vi "MFC-RT.vi"(0 "MFC":string(combo)="27", 5 "Set Point\n(SCCM)":dbl(knob) min=0.0 max=5000.0 step=1.0 scale=0.0..5000.0) -> ()   [LabVIEW 2011]
panel:
  out "SCCM":dbl=500.0
  in  "stop":bool
  in  "Full Scale":dbl=24576.0
  out "Pressure\n(%)":dbl(slide) scale=0.0..133.0
  out "Flow\n(SCCM)":dbl(slide) scale=0.0..6650.0
  out "Valve":i16
  out "Active Instance":i8
  out "Manufacturer Specific Warnings":bool caption="Boolean"
  out "Device Profice Specific Warnings":bool caption="Boolean"
  out "Common Warnings":bool caption="Boolean"
  out "0":bool caption="Boolean"
  out "Manufactuer Specific Alarms":bool caption="Boolean"
  out "1 (Extended Reporting Enabled)":bool caption="Boolean"
  out "Device Profile Specific Alarms":bool caption="Boolean"
  out "Common Alarms":bool caption="Boolean"
  # "0    -  24576\n   0% to  100%\n\n\n 24577  - 27033\n100+% to 110%\n\n\n 27034  -  32767\n110+% to 133%"
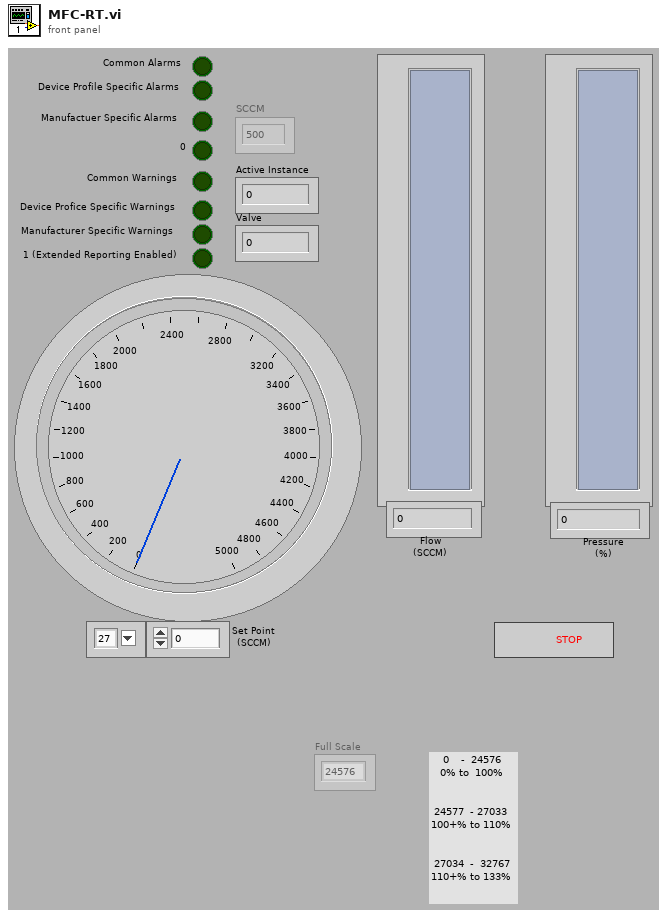
[diagram p1: front panel]
types:
  T1 = enum16{"No dialog", "OK message", "Continue or stop message", "OK message with warnings", "Continue or stop message with warnings"}
  T2 = enum16{"Read", "Write", "ReadWrite", "BufferedRead", "BufferedReadWrite"}
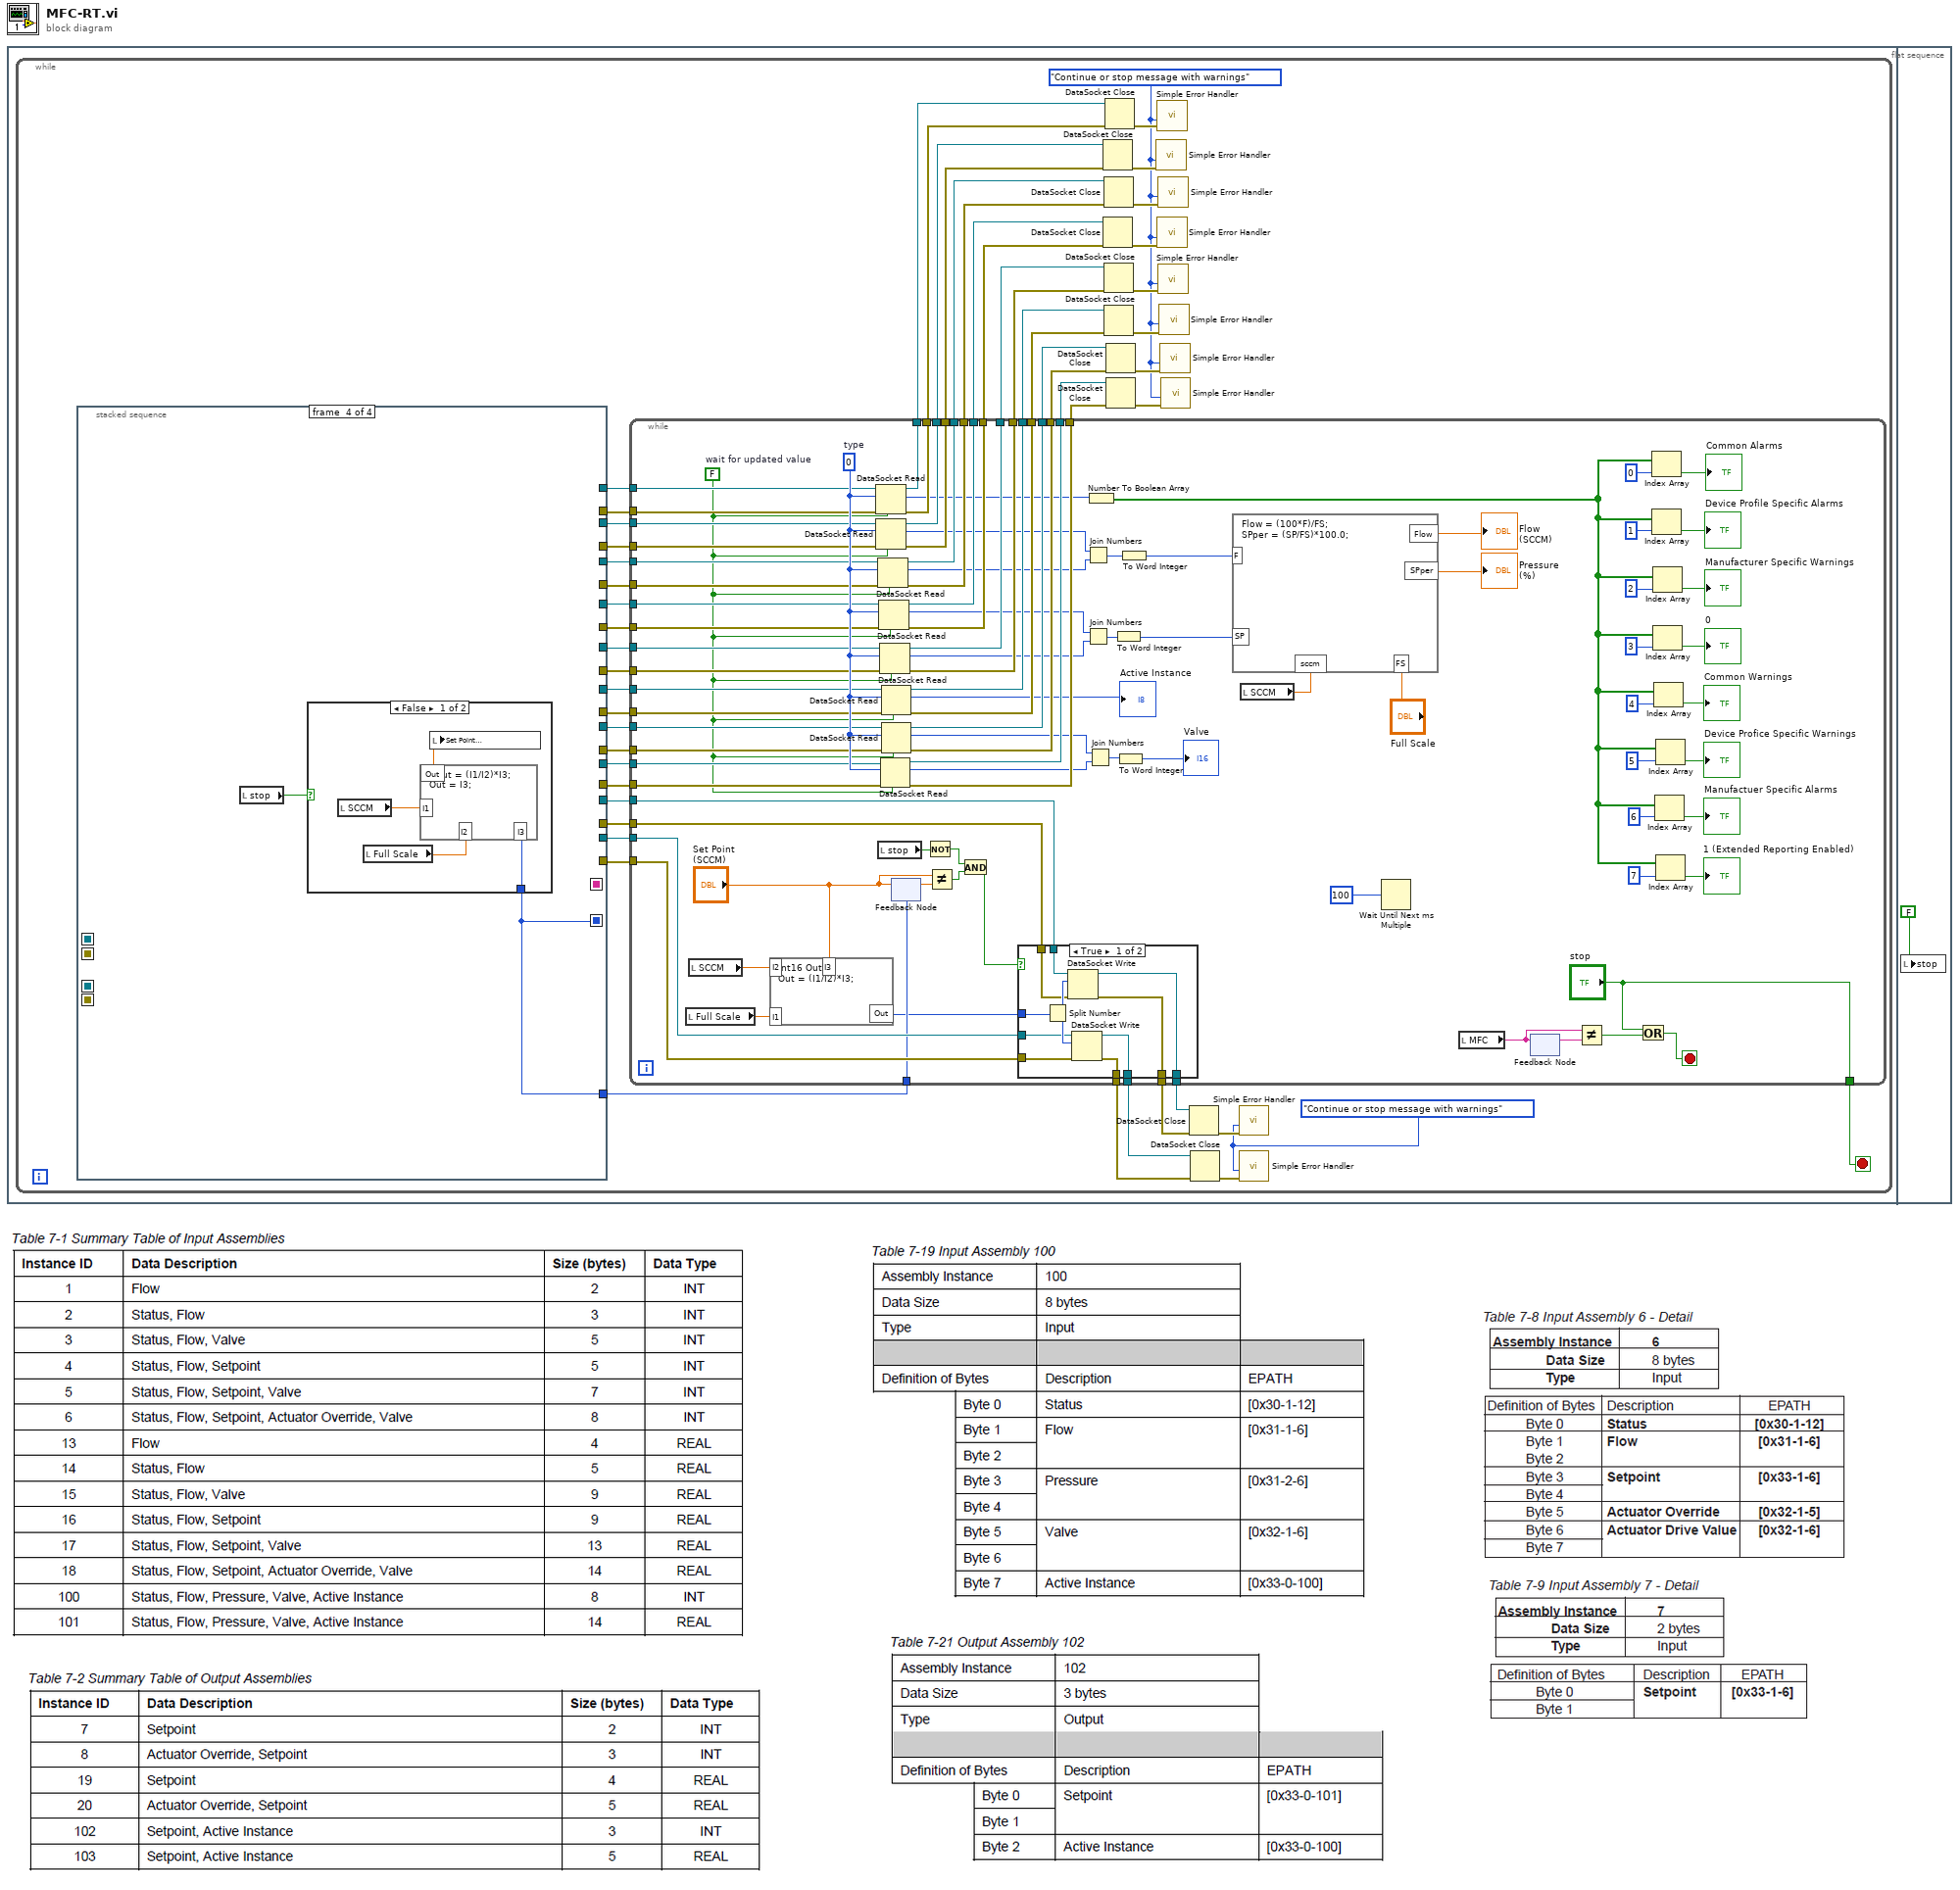
[diagram p0: block diagram]
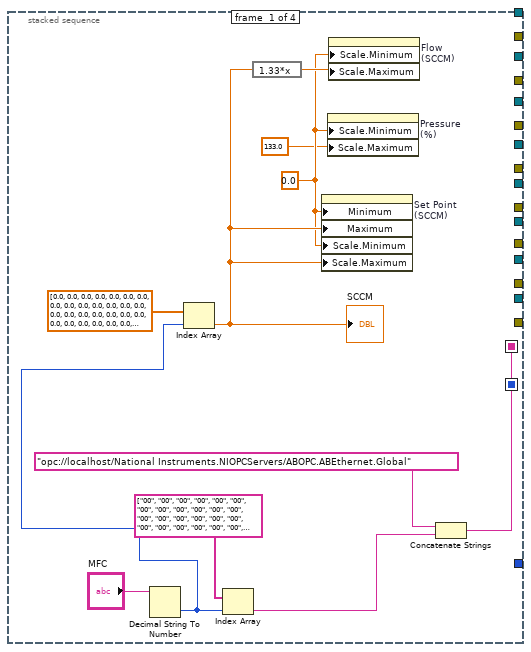
[diagram p2: hidden frame]
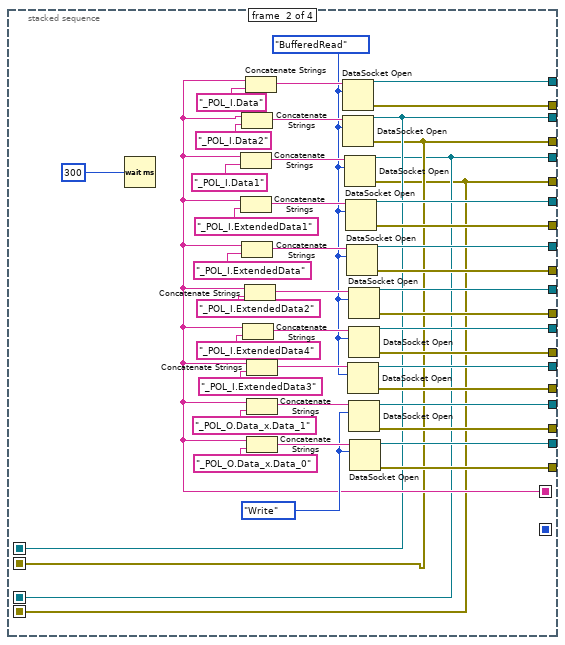
[diagram p3: hidden frame]
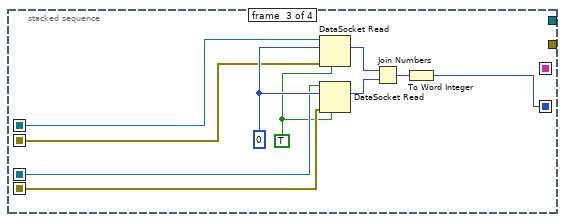
[diagram p4: hidden frame]
diagram:
  n1 = flat-sequence {
    frame #0 {
      n2 = while {
        stop <- w1 stop-if-true
        w7 = T1."Continue or stop message with warnings"
        w30 = T1."Continue or stop message with warnings"
        n3 = stacked-sequence {
          seq-local: [_ w68 _ _] -> [_ _ w115 _]
          seq-local: [_ w69 _ _] -> [_ _ w112 _]
          seq-local: [_ w66 _ _] -> [_ _ w114 _]
          seq-local: [_ w67 _ _] -> [_ _ w113 _]
          seq-local: [w62 _ _ _] -> [_ w71 _ _]
          seq-local: [_ _ w110 _] -> [_ _ _ w120]
          tunnel: [_ w108 _ _] -> w54
          tunnel: [_ w109 _ _] -> w53
          tunnel: [_ w107 _ _] -> w52
          tunnel: [_ w106 _ _] -> w51
          tunnel: [_ w81 _ _] -> w50
          tunnel: [_ w80 _ _] -> w49
          tunnel: [_ w79 _ _] -> w48
          tunnel: [_ w78 _ _] -> w47
          tunnel: [_ w77 _ _] -> w46
          tunnel: [_ w76 _ _] -> w45
          tunnel: [_ w66 _ _] -> w44
          tunnel: [_ w67 _ _] -> w43
          tunnel: [_ w68 _ _] -> w42
          tunnel: [_ w69 _ _] -> w41
          tunnel: [_ w87 _ _] -> w40
          tunnel: [_ w86 _ _] -> w39
          tunnel: [_ w75 _ _] -> w6
          tunnel: [_ w72 _ _] -> w5
          tunnel: [_ w74 _ _] -> w4
          tunnel: [_ w73 _ _] -> w3
          tunnel: [_ _ _ w120] -> w2
          frame #0 {
            w56 = 0.0
            n4 = Decimal String To Number(string="MFC") -> (number=w58:i32)  [unwired: 2 in, 1 out]
            n5 = Index Array(array=dbl[] [0.0, 0.0, 0.0, 0.0, 0.0, 0.0, 0.0, 0.0, 0.0, 0.0, 0.0, 0.0, 0.0, 0.0, 0.0, 0.0, 0.0, 0.0, 0.0, 0.0, 0.0, 0.0, 0.0, 0.0, 0.0, 0.0, 0.0, 5000.0, 5000.0, 5000.0], index=w58) -> (element=w59:dbl)
            "SCCM" <- w59
            n6 = Index Array(array=string[] ["00", "00", "00", "00", "00", "00", "00", "00", "00", "00", "00", "00", "00", "00", "00", "00", "00", "00", "00", "00", "00", "00", "00", "00", "00", "00", "00", ".Dnet_A_N53", ".Dnet_A_N54", ".Dnet_A_N49"], index=w58) -> (element=w63:string)
            n7 = expression code="1.33*x"(w59) -> (w57:dbl)
            n8 = property on="Set Point\n(SCCM)" class="Knob (strict)"("Minimum"=w56, "Maximum"=w59, "Scale.Minimum"=w56, "Scale.Maximum"=w59) -> ()  [unwired: 2 in, 2 out]
            n9 = property on="Pressure\n(%)" class="Slide (strict)"("Scale.Minimum"=w56, "Scale.Maximum"=133.0) -> ()  [unwired: 2 in, 2 out]
            n10 = property on="Flow\n(SCCM)" class="Slide (strict)"("Scale.Minimum"=w56, "Scale.Maximum"=w57) -> ()  [unwired: 2 in, 2 out]
            n11 = Concatenate Strings("opc://localhost/National Instruments.NIOPCServers/ABOPC.ABEthernet.Global", w63) -> (w62:string)
          }
          frame #1 {
            w82 = T2."Write" ("mode")
            w85 = T2."BufferedRead" ("mode")
            n12 = Wait (ms)(milliseconds to wait=u32 300) -> ()  [unwired: 1 out]
            n13 = Concatenate Strings(w71, "_POL_I.Data1") -> (w93:string)
            n14 = Concatenate Strings(w71, "_POL_I.ExtendedData1") -> (w92:string)
            n15 = Concatenate Strings(w71, "_POL_I.Data2") -> (w94:string)
            n16 = Concatenate Strings(w71, "_POL_I.ExtendedData") -> (w91:string)
            n17 = Concatenate Strings(w71, "_POL_I.ExtendedData4") -> (w89:string)
            n18 = Concatenate Strings(w71, "_POL_I.ExtendedData2") -> (w90:string)
            n19 = Concatenate Strings(w71, "_POL_I.Data") -> (w95:string)
            n20 = Concatenate Strings(w71, "_POL_I.ExtendedData3") -> (w88:string)
            n21 = Concatenate Strings(w71, "_POL_O.Data_x.Data_1") -> (w83:string)
            n22 = Concatenate Strings(w71, "_POL_O.Data_x.Data_0") -> (w84:string)
            n23 = DataSocket Open(10:w85, 11:w95) -> (0:w87:errorcluster, 3:w86:refnum<k13>)  [unwired: 2 in]
            n24 = DataSocket Open(10:w85, 11:w94) -> (0:w68:errorcluster, 3:w69:refnum<k13>)  [unwired: 2 in]
            n25 = DataSocket Open(10:w85, 11:w93) -> (0:w66:errorcluster, 3:w67:refnum<k13>)  [unwired: 2 in]
            n26 = DataSocket Open(10:w85, 11:w92) -> (0:w109:errorcluster, 3:w108:refnum<k13>)  [unwired: 2 in]
            n27 = DataSocket Open(10:w85, 11:w91) -> (0:w106:errorcluster, 3:w107:refnum<k13>)  [unwired: 2 in]
            n28 = DataSocket Open(10:w85, 11:w88) -> (0:w80:errorcluster, 3:w81:refnum<k13>)  [unwired: 2 in]
            n29 = DataSocket Open(10:w85, 11:w90) -> (0:w77:errorcluster, 3:w76:refnum<k13>)  [unwired: 2 in]
            n30 = DataSocket Open(10:w85, 11:w89) -> (0:w79:errorcluster, 3:w78:refnum<k13>)  [unwired: 2 in]
            n31 = DataSocket Open(10:w82, 11:w83) -> (0:w72:errorcluster, 3:w75:refnum<k13>)  [unwired: 2 in]
            n32 = DataSocket Open(10:w82, 11:w84) -> (0:w73:errorcluster, 3:w74:refnum<k13>)  [unwired: 2 in]
          }
          frame #2 {
            w111 = TRUE
            w116 = i8 0
            n33 = DataSocket Read(6:w111, 8:w115, 10:w116, 11:w112) -> (2:w118:i8)  [unwired: 1 in, 6 out]
            n34 = DataSocket Read(6:w111, 8:w114, 10:w116, 11:w113) -> (2:w119:i8)  [unwired: 1 in, 6 out]
            n35 = Join Numbers(hi=w118, lo=w119) -> ((hi.lo)=w117:u16)
            n36 = To Word Integer(number=w117) -> (16bit integer=w110:i16)
          }
          frame #3 {
            n37 = local read "stop"() -> (w121:bool)
            n38 = case shown="False" w121 {
              tunnel: w120 -> [w122 _]
              frame False {
                n39 = local read "SCCM"() -> (w123:dbl)
                n40 = local read "Full Scale"() -> (w125:dbl)
                n41 = formula code="//Out = (I1/I2)*I3;\nOut = I3;"("I1"=w123, "I2"=w125, "I3"=w122) -> ("Out"=w124:dbl)
                n42 = local write "Set Point\n(SCCM)"(w124) -> ()
              }
              frame True {
              }
            }
          }
        }
        n43 = while {
          tunnel: w50 -> [w195]
          tunnel: w49 -> [w194]
          tunnel: w48 -> [w193]
          tunnel: w47 -> [w192]
          tunnel: w46 -> [w191]
          tunnel: w45 -> [w190]
          tunnel: w51 -> [w189]
          tunnel: w52 -> [w188]
          tunnel: w53 -> [w187]
          tunnel: w54 -> [w186]
          tunnel: w44 -> [w185]
          tunnel: w43 -> [w184]
          tunnel: w42 -> [w183]
          tunnel: w41 -> [w182]
          tunnel: w40 -> [w181]
          tunnel: w39 -> [w180]
          tunnel: [w179] -> w29
          tunnel: [w178] -> w28
          tunnel: [w177] -> w27
          tunnel: [w176] -> w26
          tunnel: [w175] -> w25
          tunnel: [w174] -> w24
          tunnel: [w173] -> w23
          tunnel: [w172] -> w22
          tunnel: [w171] -> w21
          tunnel: [w170] -> w20
          tunnel: [w169] -> w19
          tunnel: [w168] -> w18
          tunnel: [w167] -> w17
          tunnel: [w166] -> w16
          tunnel: [w165] -> w15
          tunnel: [w164] -> w14
          tunnel: [w161] -> w11
          tunnel: [w160] -> w10
          tunnel: [w159] -> w9
          tunnel: [w158] -> w8
          tunnel: w6 -> [w157]
          tunnel: w5 -> [w156]
          tunnel: w4 -> [w155]
          tunnel: w3 -> [w154]
          tunnel: w2 -> [w153]
          tunnel: ["stop"] -> w1
          stop <- w197 stop-if-true
          w162 = FALSE  # wait for updated value
          w218 = i8 0  # type
          n44 = local read "Full Scale"() -> (w138:dbl)
          n45 = local read "SCCM"() -> (w134:dbl)
          n46 = formula code="int16 Out;\nOut = (I1/I2)*I3;"("I3"="Set Point\n(SCCM)", "I1"=w138, "I2"=w134) -> ("Out"=w137:i16)
          n47 = DataSocket Read(6:w162, 8:w181, 10:w218, 11:w180) -> (0:w175:errorcluster, 2:w140:i8, 3:w176:refnum<k13>)  [unwired: 1 in, 4 out]
          n48 = DataSocket Read(6:w162, 8:w183, 10:w218, 11:w182) -> (0:w173:errorcluster, 2:w141:i8, 3:w174:refnum<k13>)  [unwired: 1 in, 4 out]
          n49 = DataSocket Read(6:w162, 8:w185, 10:w218, 11:w184) -> (0:w171:errorcluster, 2:w142:i8, 3:w172:refnum<k13>)  [unwired: 1 in, 4 out]
          n50 = local read "stop"() -> (w151:bool)
          n51 = DataSocket Read(6:w162, 8:w187, 10:w218, 11:w186) -> (0:w169:errorcluster, 2:w143:i8, 3:w170:refnum<k13>)  [unwired: 1 in, 4 out]
          n52 = DataSocket Read(6:w162, 8:w189, 10:w218, 11:w188) -> (0:w166:errorcluster, 2:w144:i8, 3:w164:refnum<k13>)  [unwired: 1 in, 4 out]
          n53 = DataSocket Read(6:w162, 8:w194, 10:w218, 11:w195) -> (0:w179:errorcluster, 2:w147:i8, 3:w178:refnum<k13>)  [unwired: 1 in, 4 out]
          n54 = DataSocket Read(6:w162, 8:w191, 10:w218, 11:w190) -> (0:w168:errorcluster, 2:→"Active Instance":i8, 3:w165:refnum<k13>)  [unwired: 1 in, 4 out]
          n55 = DataSocket Read(6:w162, 8:w193, 10:w218, 11:w192) -> (0:w177:errorcluster, 2:w146:i8, 3:w167:refnum<k13>)  [unwired: 1 in, 4 out]
          n56 = feedback #1(w153) -> (w152:dbl)
          n57 = feedback-in #1("Set Point\n(SCCM)") -> ()
          n58 = Not(x=w151) -> (.not. x?=w148:bool)
          n59 = Not Equal?(x="Set Point\n(SCCM)", y=w152) -> (x != y?=w149:bool)
          n60 = And(x=w148, y=w149) -> (x .and. y?=w150:bool)
          n61 = case shown="True" w150 {
            tunnel: w137 -> [w227 _]
            tunnel: [w226 w230] -> w161
            tunnel: [w225 w231] -> w160
            tunnel: [w224 w232] -> w159
            tunnel: [w223 w233] -> w158
            tunnel: w157 -> [w222 w233]
            tunnel: w156 -> [w221 w232]
            tunnel: w155 -> [w220 w231]
            tunnel: w154 -> [w219 w230]
            frame True {
              n62 = Split Number(x=w227) -> (hi(x)=w229:u8, lo(x)=w228:u8)
              n63 = DataSocket Write(8:w221, 10:w229, 11:w222) -> (0:w224:errorcluster, 3:w223:refnum<k13>)  [unwired: 1 in, 1 out]
              n64 = DataSocket Write(8:w219, 10:w228, 11:w220) -> (0:w226:errorcluster, 3:w225:refnum<k13>)  [unwired: 1 in, 1 out]
            }
            frame False {
            }
          }
          n65 = Join Numbers(hi=w141, lo=w142) -> ((hi.lo)=w200:u16)
          n66 = Join Numbers(hi=w143, lo=w144) -> ((hi.lo)=w201:u16)
          n67 = Join Numbers(hi=w146, lo=w147) -> ((hi.lo)=w136:u16)
          n68 = Number To Boolean Array(number=w140) -> (Boolean array=w199:bool[])
          n69 = To Word Integer(number=w201) -> (16bit integer=w132:i16)
          n70 = To Word Integer(number=w136) -> (16bit integer=→"Valve":i16)
          n71 = To Word Integer(number=w200) -> (16bit integer=w133:i16)
          n72 = local read "SCCM"() -> (w131:dbl)
          n73 = formula code="Flow = (100*F)/FS;\nSPper = (SP/FS)*100.0;"("FS"="Full Scale", "F"=w133, "SP"=w132, "sccm"=w131) -> ("Flow"=→"Flow\n(SCCM)":dbl, "SPper"=→"Pressure\n(%)":dbl)
          n74 = Wait Until Next ms Multiple(millisecond multiple=u32 100) -> ()  [unwired: 1 out]
          n75 = local read "MFC"() -> (w196:string)
          n76 = feedback #2() -> (w198:string)  [unwired: 1 in]
          n77 = feedback-in #2(w196) -> ()
          n78 = Not Equal?(x=w196, y=w198) -> (x != y?=w127:bool)
          n79 = Or(x="stop", y=w127) -> (x .or. y?=w197:bool)
          n80 = Index Array(array=w199, index=0) -> (element=→"Common Alarms":bool)
          n81 = Index Array(array=w199, index=1) -> (element=→"Device Profile Specific Alarms":bool)
          n82 = Index Array(array=w199, index=2) -> (element=→"Manufacturer Specific Warnings":bool)
          n83 = Index Array(array=w199, index=3) -> (element=→"0":bool)
          n84 = Index Array(array=w199, index=4) -> (element=→"Common Warnings":bool)
          n85 = Index Array(array=w199, index=6) -> (element=→"Manufactuer Specific Alarms":bool)
          n86 = Index Array(array=w199, index=5) -> (element=→"Device Profice Specific Warnings":bool)
          n87 = Index Array(array=w199, index=7) -> (element=→"1 (Extended Reporting Enabled)":bool)
        }
        n88 = DataSocket Close(8:w23, 11:w24) -> (0:w32:errorcluster)  [unwired: 1 in, 1 out]
        n89 = DataSocket Close(8:w19, 11:w20) -> (0:w34:errorcluster)  [unwired: 1 in, 1 out]
        n90 = DataSocket Close(8:w21, 11:w22) -> (0:w33:errorcluster)  [unwired: 1 in, 1 out]
        n91 = DataSocket Close(8:w16, 11:w14) -> (0:w35:errorcluster)  [unwired: 1 in, 1 out]
        n92 = DataSocket Close(8:w18, 11:w15) -> (0:w36:errorcluster)  [unwired: 1 in, 1 out]
        n93 = DataSocket Close(8:w25, 11:w26) -> (0:w31:errorcluster)  [unwired: 1 in, 1 out]
        n94 = DataSocket Close(8:w27, 11:w17) -> (0:w37:errorcluster)  [unwired: 1 in, 1 out]
        n95 = DataSocket Close(8:w29, 11:w28) -> (0:w38:errorcluster)  [unwired: 1 in, 1 out]
        n96 = call <vilib>:"Simple Error Handler.vi"("type of dialog (OK msg:1)"=w30, "error in (no error)"=w32) -> ()  [unwired: 3 in, 5 out]
        n97 = call <vilib>:"Simple Error Handler.vi"("type of dialog (OK msg:1)"=w30, "error in (no error)"=w31) -> ()  [unwired: 3 in, 5 out]
        n98 = call <vilib>:"Simple Error Handler.vi"("type of dialog (OK msg:1)"=w30, "error in (no error)"=w34) -> ()  [unwired: 3 in, 5 out]
        n99 = call <vilib>:"Simple Error Handler.vi"("type of dialog (OK msg:1)"=w30, "error in (no error)"=w33) -> ()  [unwired: 3 in, 5 out]
        n100 = call <vilib>:"Simple Error Handler.vi"("type of dialog (OK msg:1)"=w30, "error in (no error)"=w35) -> ()  [unwired: 3 in, 5 out]
        n101 = call <vilib>:"Simple Error Handler.vi"("type of dialog (OK msg:1)"=w30, "error in (no error)"=w36) -> ()  [unwired: 3 in, 5 out]
        n102 = call <vilib>:"Simple Error Handler.vi"("type of dialog (OK msg:1)"=w30, "error in (no error)"=w37) -> ()  [unwired: 3 in, 5 out]
        n103 = call <vilib>:"Simple Error Handler.vi"("type of dialog (OK msg:1)"=w30, "error in (no error)"=w38) -> ()  [unwired: 3 in, 5 out]
        n104 = DataSocket Close(8:w9, 11:w8) -> (0:w12:errorcluster)  [unwired: 1 in, 1 out]
        n105 = DataSocket Close(8:w11, 11:w10) -> (0:w13:errorcluster)  [unwired: 1 in, 1 out]
        n106 = call <vilib>:"Simple Error Handler.vi"("type of dialog (OK msg:1)"=w7, "error in (no error)"=w12) -> ()  [unwired: 3 in, 5 out]
        n107 = call <vilib>:"Simple Error Handler.vi"("type of dialog (OK msg:1)"=w7, "error in (no error)"=w13) -> ()  [unwired: 3 in, 5 out]
      }
    }
    frame #1 {
      n108 = local write "stop"(FALSE) -> ()
    }
  }
